vi "Get Distance.vi"(10 "Starting value":dbl, 11 "PotDevRef":T1) -> (3 "Distance":dbl)   [LabVIEW 2015]
uses:
  <vilib>/Rock Robotics/WPI/Potentiometer/WPI_PotentiometerDevRef.ctl
  <vilib>/Rock Robotics/SystemInterfaces/AI/FPGA_AIChannel.ctl
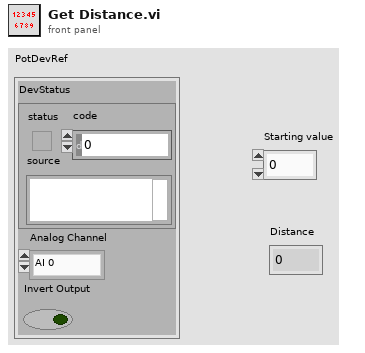
[diagram p1: front panel]
types:
  T1 = typedef "WPI_PotentiometerDevRef.ctl" = cluster{"DevStatus":errorcluster, "Analog Channel":T2, "Invert Output":bool}
  T2 = typedef "FPGA_AIChannel.ctl" = enum8{"AI 0", "AI 1", "AI 2", "AI 3", "AI MXP 0", "AI MXP 1", "AI MXP 2", "AI MXP 3", "Invalid"}
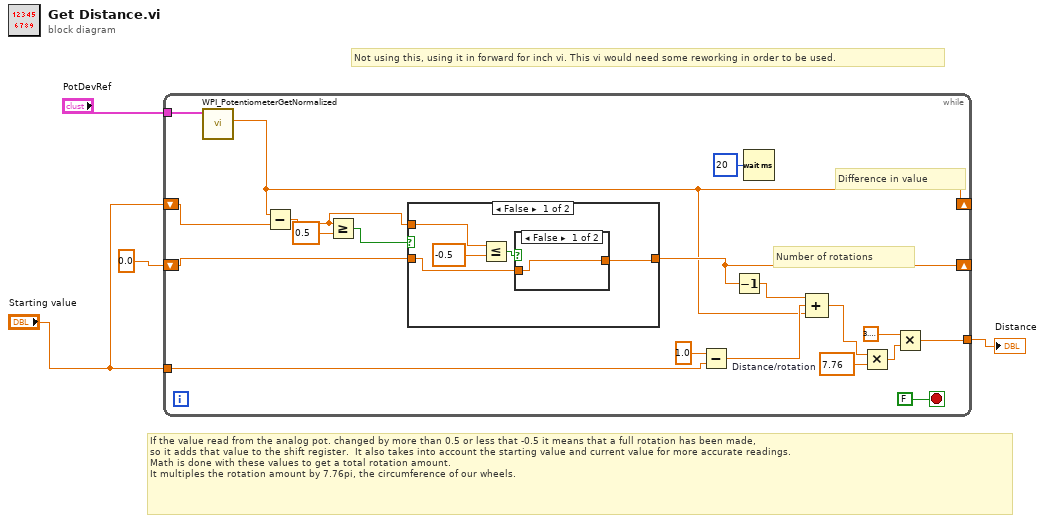
[diagram p0: block diagram]
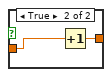
[diagram p2: hidden frame]
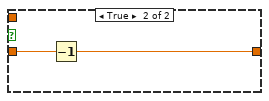
[diagram p3: hidden frame]
diagram:
  # "Not using this, using it in forward for inch vi. This vi would need some reworking in order to be used."
  # "If the value read from the analog pot. changed by more than 0.5 or less that -0.5 it means that a full rotation has been made, \nso it adds that value to the shift register.  It also takes into account the starting value and current value for more accurate readings.\nMath is done with these values to get a total rotation amount.\nIt multiples the rotation amount by 7.76pi, the circumference of our wheels."
  n1 = while {
    shift-right: [w11] -> _
    shift-left: "Starting value" -> [w21]
    tunnel: "PotDevRef" -> [w23]
    shift-right: [w14] -> _
    shift-left: 0.0 -> [w18]
    tunnel: "Starting value" -> [w15]
    tunnel: [w5] -> w2
    stop <- FALSE stop-if-true
    w10 = 7.76  # Distance/rotation
    # "Number of rotations"
    # "Difference in value"
    n2 = call <vilib>:"WPI_PotentiometerGetNormalized.vi"("PotDevRef"=w23) -> ("Normalized Value"=w11:dbl)  [unwired: 8 in, 2 out]
    n3 = Subtract(x=w11, y=w21) -> (x-y=w17:dbl)
    n4 = Greater Or Equal?(x=w17, y=0.5) -> (x >= y?=w19:bool)
    n5 = case shown="False" w19 {
      tunnel: [w24 w33] -> w14
      tunnel: w18 -> [w25 w32]
      tunnel: w17 -> [w28 _]
      frame False {
        n6 = Less Or Equal?(x=w28, y=-0.5) -> (x <= y?=w26:bool)
        n7 = case shown="False" w26 {
          tunnel: w25 -> [w29 w31]
          tunnel: [w29 w30] -> w24
          frame False {
          }
          frame True {
            n8 = Increment(x=w31) -> (x+1=w30:dbl)
          }
        }
      }
      frame True {
        n9 = Decrement(x=w32) -> (x-1=w33:dbl)
      }
    }
    n10 = Subtract(x=1.0, y=w15) -> (x-y=w12:dbl)
    n11 = Decrement(x=w14) -> (x-1=w13:dbl)
    n12 = Wait (ms)(milliseconds to wait=u32 20) -> ()  [unwired: 1 out]
    n13 = Compound Arithmetic op=ADD(w13, w12, w11) -> (w9:dbl)
    n14 = Multiply(x=w9, y=w10) -> (x*y=w7:dbl)
    n15 = Multiply(x=3.141592653589793, y=w7) -> (x*y=w5:dbl)
  }
  "Distance" <- w2
